vi "gas flow action stack.vi"(7 "action":T2, 9 "selector in":T1=enum."stop UP/DOWN", 11 "command stack":T1[](array[typedef])) -> (1 "selector out":T1=enum."stop UP/DOWN", 2 "stack is empty ?":bool, 3 "command stack out":T1[](array[typedef]))   [LabVIEW 2015]
uses:
  stack action -- control.ctl
  gas flow controller action.ctl
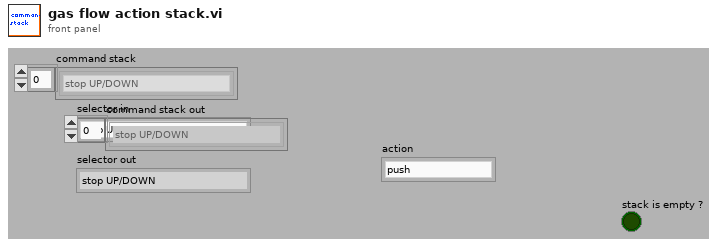
[diagram p1: front panel]
types:
  T1 = typedef "gas flow controller action.ctl" = enum16{"check", "force UP", "stop UP/DOWN", "force DOWN", "init", "set gas to", "turn off", "turn on", "idle", "update parameters", "parse", "set gas"}
  T2 = typedef "stack action -- control.ctl" = enum16{"push", "pop", "check", "init"}
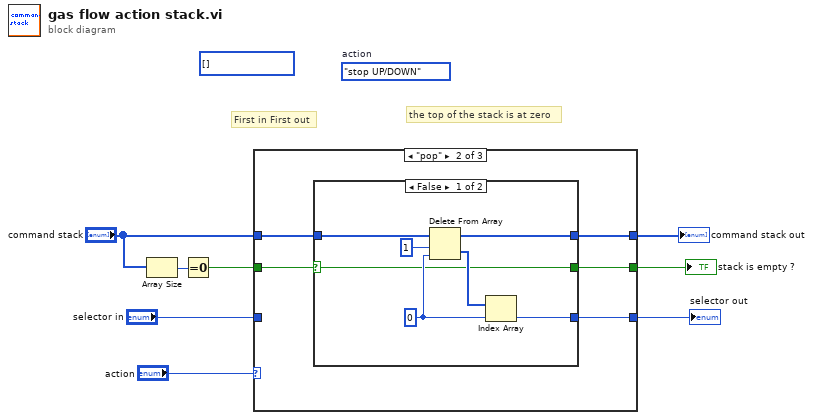
[diagram p0: block diagram]
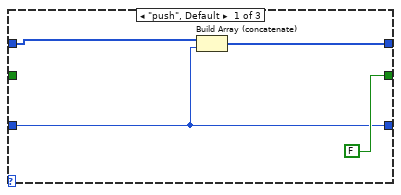
[diagram p2: hidden frame]
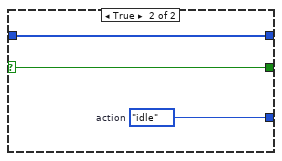
[diagram p3: hidden frame]
diagram:
  (unwired) gas_flow_controller_action."stop UP/DOWN"  # action
  (unwired) T1[] [] items=["check", "force UP", "stop UP/DOWN", "force DOWN", "init", "set gas to", "turn off", "turn on", "idle", "update parameters", "parse", "set gas"]
  # "First in First out"
  # "the top of the stack is at zero"
  n1 = Array Size(array="command stack") -> (size(s)=w8:i32)
  n2 = Equal To 0?(x=w8) -> (x = 0?=w7:bool)
  n3 = case shown="\"pop\"" "action" {
    tunnel: [w12 w17 w28] -> w2
    tunnel: "command stack" -> [w10 w16 w28]
    tunnel: w7 -> [_ w15 w30]
    tunnel: [w9 w14 w29] -> w1
    tunnel: [FALSE w13 w30] -> w5
    tunnel: "selector in" -> [w9 _ w29]
    frame "push", Default {
      n4 = Build Array (concatenate)(w10, w9) -> (w12:T1[])
    }
    frame "pop" {
      n5 = case shown="False" w15 {
        selector: w15 -> [w18 w26]
        tunnel: [w24 w27] -> w17
        tunnel: w16 -> [w23 w27]
        tunnel: [w19 w25] -> w14
        tunnel: [w18 w26] -> w13
        frame False {
          w20 = 0
          n6 = Delete From Array(array=w23, length=1, index=w20) -> (deleted portion=w21:T1[], array with subset deleted=w24:T1[])
          n7 = Index Array(array=w21, index=w20) -> (element=w19:T1)
        }
        frame True {
          w25 = gas_flow_controller_action."idle"  # action
        }
      }
    }
    frame "check" {
    }
  }
  "stack is empty ?" <- w5
  "command stack out" <- w2
  "selector out" <- w1
